vi "TCP Server - VI Tree.vi"() -> ()   [LabVIEW 2020]
uses:
  _Data Structures/TCP Server Connection Process Data Cluster.ctl
  JKI TCP Server.lvclass
panel:
  in  "TCP Server":refnum<class "JKI TCP Server.lvclass">
  in  "Connection Data":T1
  # "TCP Server VI Tree"
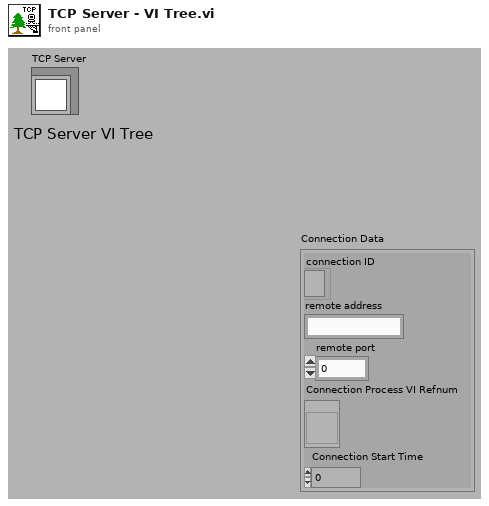
[diagram p1: front panel]
types:
  T1 = typedef "JKI TCP Server.lvclass/TCP Server Connection Process Data Cluster.ctl" = cluster{"connection ID":refnum<k5>, "remote address":string, "remote port":u16, "Connection Process VI Refnum":refnum<vi>, "Connection Start Time":u32}
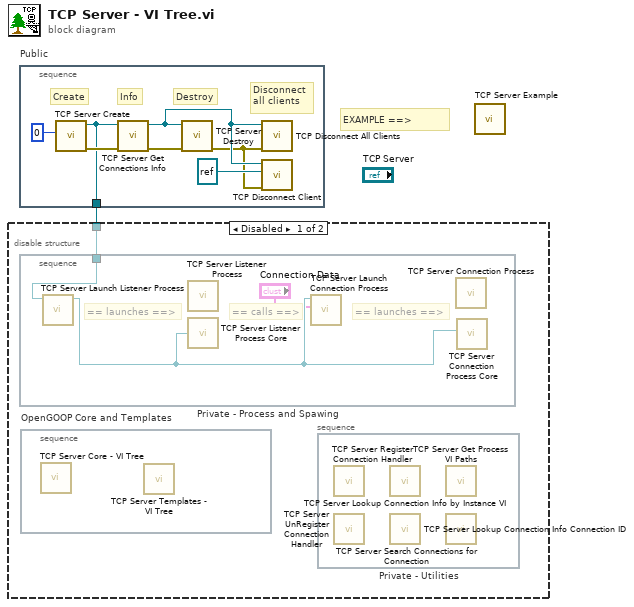
[diagram p0: block diagram]
diagram:
  # "EXAMPLE ==>"
  n1 = stacked-sequence "Public" {
    tunnel: [w5] -> w1
    frame #0 {
      # "Disconnect\nall clients"
      # "Destroy"
      # "Info"
      # "Create"
      n2 = call "TCP Server Create.vi"("port"=u16 0) -> ("error out"=w7:errorcluster, "TCP Server"=w5:refnum<class "JKI TCP Server.lvclass">)  [unwired: 9 in]
      n3 = call "TCP Server Get Connections Info.vi"("error in (no error)"=w7, "TCP Server"=w5) -> ("error out"=w6:errorcluster, "TCP Server out"=w4:refnum<class "JKI TCP Server.lvclass">)  [unwired: 5 in, 3 out]
      n4 = call "TCP Server Destroy.vi"("error in (no error)"=w6, "TCP Server"=w4) -> ("error out"=w2:errorcluster)  [unwired: 9 in]
      n5 = call "TCP Disconnect All Clients.vi"("error in (no error)"=w2, "TCP Server"=w4) -> ()  [unwired: 8 in, 2 out]
      n6 = call "TCP Disconnect Client.vi"("error in"=w2, "connection ID"=refnum<k5> refnum, "TCP Server"=w4) -> ()  [unwired: 8 in, 1 out]
    }
  }
  n7 = disable-structure shown="Disabled" {
    disable-tunnel: w1 -> [w9 _]
    frame Disabled {
      n8 = stacked-sequence "Private - Process and Spawing" {
        tunnel: w9 -> [w10]
        frame #0 {
          # "== calls ==>"
          # "== launches ==>"
          # "== launches ==>"
          n9 = call "TCP Server Launch Listener Process.vi"("RefNum"=w10) -> ("dup RefNum"=w12:refnum<class "JKI TCP Server.lvclass">)  [unwired: 9 in, 1 out]
          n10 = call "TCP Server Listener Process.vi"() -> ()  [unwired: 1 in]
          n11 = call "TCP Server Listener Process Core.vi"("TCP Server RefNum"=w12) -> ()
          n12 = call "TCP Server Launch Connection Process.vi"("Connection Data"="Connection Data", "TCP Server RefNum"=w12) -> ()  [unwired: 9 in, 1 out]
          n13 = call "TCP Server Connection Process.vi"() -> ()  [unwired: 1 in]
          n14 = call "TCP Server Connection Process Core.vi"("TCP Server Refnum"=w12) -> ()  [unwired: 11 in]
        }
      }
      n15 = stacked-sequence "OpenGOOP Core and Templates" {
        frame #0 {
          n16 = call "TCP Server Core - VI Tree.vi"() -> ()  [unwired: 1 in]
          n17 = call "TCP Server Templates - VI Tree.vi"() -> ()  [unwired: 1 in]
        }
      }
      n18 = stacked-sequence "Private - Utilities" {
        frame #0 {
          n19 = call "TCP Server Register Connection Handler.vi"() -> ()  [unwired: 9 in, 3 out]
          n20 = call "TCP Server UnRegister Connection Handler.vi"() -> ()  [unwired: 9 in, 3 out]
          n21 = call "TCP Server Lookup Connection Info by Instance VI.vi"() -> ()  [unwired: 6 in, 6 out]
          n22 = call "TCP Server Lookup Connection Info Connection ID.vi"() -> ()  [unwired: 10 in, 2 out]
          n23 = call "TCP Server Get Process VI Paths.vi"() -> ()  [unwired: 1 out]
          n24 = call "TCP Server Search Connections for Connection.vi"() -> ()  [unwired: 3 in, 3 out]
        }
      }
    }
    frame Enabled {
    }
  }
  n25 = call "TCP Server Example.vi"() -> ()  [unwired: 1 in]
